vi "Exponential Joystick Control.vi"(9 "z exponent":dbl format="%#_13g", 10 "x & y exponent":dbl format="%#_13g", 11 "Axes Magnitudes":cluster{"X":dbl, "Y":dbl, "Z":dbl}) -> (3 "Axes Magnitudes Out":cluster{"X":dbl, "Y":dbl, "Z":dbl})   [LabVIEW 2018]
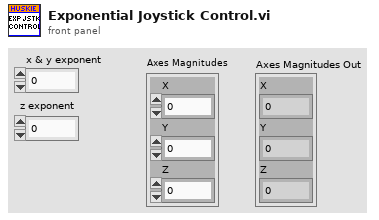
[diagram p1: front panel]
types:
  T1 = cluster{"Joystick 1 X":dbl, "Joystick 1 Y":dbl, "Joystick 2 Z":dbl}
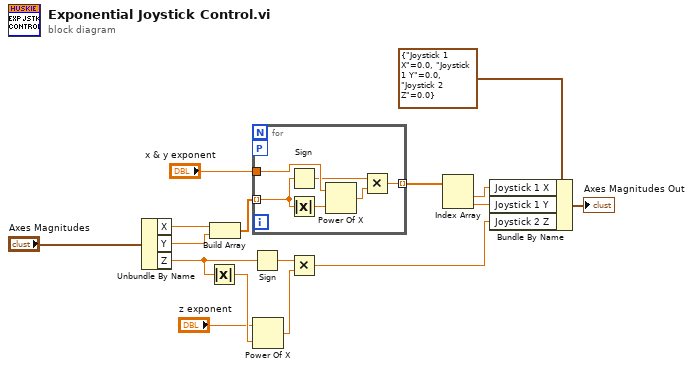
[diagram p0: block diagram]
diagram:
  n1 = Unbundle By Name("Axes Magnitudes") -> ("X"=w10:dbl, "Y"=w9:dbl, "Z"=w8:dbl)
  n2 = Absolute Value(x=w8) -> (abs(x)=w15:dbl)
  n3 = Build Array(w10, w9) -> (w11:dbl[])
  n4 = Sign(1:w8) -> (0:w16:dbl)
  n5 = for {
    tunnel: w11 -> [w19] mode=indexing
    tunnel: "x & y exponent" -> [w22]
    tunnel: [w17] -> w6 mode=indexing
    workers-P: _ -> [_]
    n6 = Sign(1:w19) -> (0:w18:dbl)
    n7 = Absolute Value(x=w19) -> (abs(x)=w20:dbl)
    n8 = Power Of X(1:w20, 2:w22) -> (0:w21:dbl)
    n9 = Multiply(x=w18, y=w21) -> (x*y=w17:dbl)
  }
  n10 = Power Of X(1:w15, 2:"z exponent") -> (0:w14:dbl)
  n11 = Multiply(x=w16, y=w14) -> (x*y=w2:dbl)
  n12 = Index Array(array=w6) -> (element #1=w5:dbl, element #2=w4:dbl)  [unwired: 2 in]
  n13 = Bundle By Name(cluster=T1 {"Joystick 1 X"=0.0, "Joystick 1 Y"=0.0, "Joystick 2 Z"=0.0} ("input cluster"), "Joystick 1 X"=w5, "Joystick 1 Y"=w4, "Joystick 2 Z"=w2) -> (→"Axes Magnitudes Out":T1)
